vi "MongoDB.CreateIndex.vi"(8 "error in (no error)":errorcluster, 10 "keyNames":string[](array[string]), 11 "MongoDB.Collection in":refnum<class "MongoDB.Collection.lvclass">) -> (0 "error out":errorcluster, 2 "Result":T1, 3 "MongoDB.Collection out":refnum<class "MongoDB.Collection.lvclass">)   [LabVIEW 2014, in "MongoDB.Collection.lvclass"]
uses:
  MongoDB.Collection.lvclass
  MongoDB.Collection.lvclass/MongoDB.Collection.ctl
  C:/Users/Richard/Documents/GitHub/mongo-labview-driver/CSharp/bin/MongoDB.Driver.Legacy.dll
  CSharp/bin/MongoDB.Driver.Legacy.dll
  C:/Users/Richard/Documents/GitHub/mongo-labview-driver/CSharp/bin/MongoDB.Driver.Core.dll
  CSharp/bin/MongoDB.Driver.Core.dll
  C:/Users/Richard/Documents/GitHub/mongo-labview-driver/CSharp/bin/MongoDB.Bson.dll
  CSharp/bin/MongoDB.Bson.dll
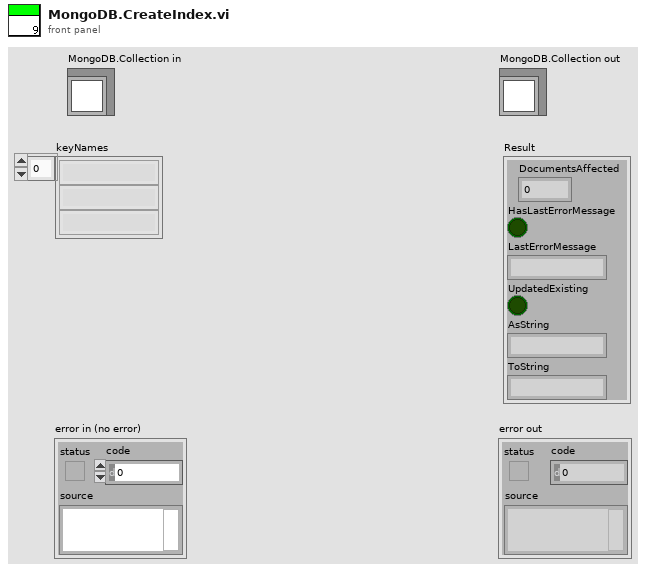
[diagram p1: front panel]
types:
  T1 = cluster{"DocumentsAffected":i64, "HasLastErrorMessage":bool, "LastErrorMessage":string, "UpdatedExisting":bool, "AsString":string, "ToString":string}
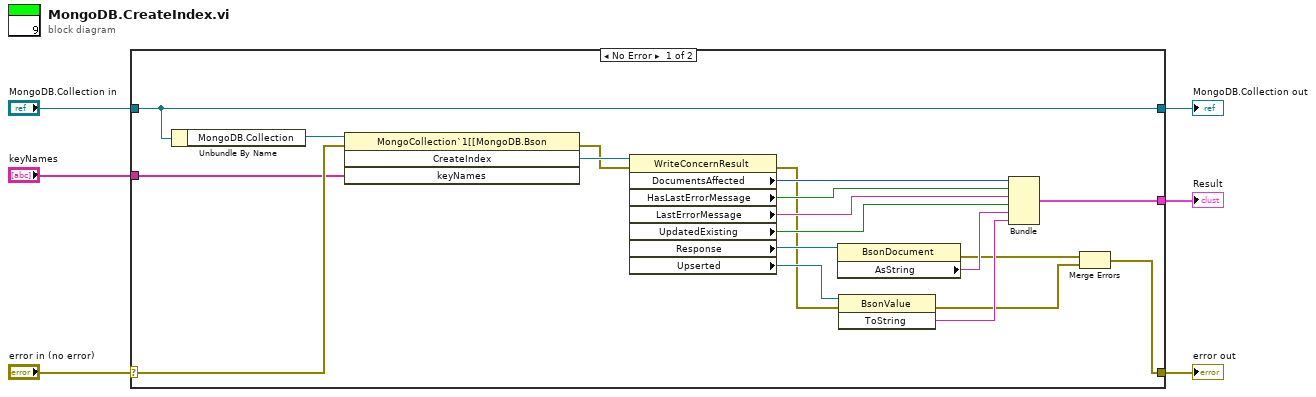
[diagram p0: block diagram]
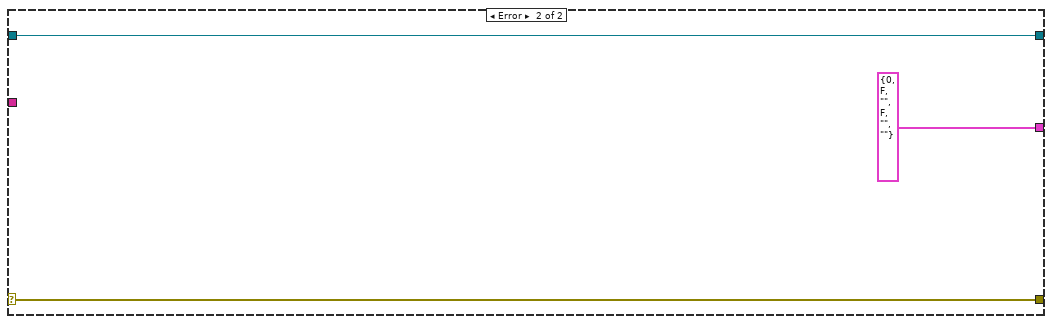
[diagram p2: hidden frame]
diagram:
  n1 = case shown="No Error" "error in (no error)" {
    selector: "error in (no error)" -> [w23 w28]
    tunnel: [w8 w28] -> w5
    tunnel: [w25 w27] -> w3
    tunnel: "MongoDB.Collection in" -> [w25 w27]
    tunnel: "keyNames" -> [w22 _]
    tunnel: [w7 T1 {"DocumentsAffected"=0, "HasLastErrorMessage"=FALSE, "LastErrorMessage"="", "UpdatedExisting"=FALSE, "AsString"="", "ToString"=""}] -> w1
    frame No Error {
      n2 = Unbundle By Name(w25) -> ("MongoDB.Collection"=w24:refnum<k24>)
      n3 = invoke class="MongoCollection`1[[MongoDB.Bson" method="CreateIndex"(reference=w24, error in=w23, "keyNames"=w22) -> (error out=w20:errorcluster, "CreateIndex"=w21:refnum<k24>)  [unwired: 1 in, 2 out]
      n4 = property class="WriteConcernResult"(reference=w21, error in=w20) -> (error out=w12:errorcluster, "DocumentsAffected"=w19:i64, "HasLastErrorMessage"=w18:bool, "LastErrorMessage"=w17:string, "UpdatedExisting"=w16:bool, "Response"=w15:refnum<k24>, "Upserted"=w13:refnum<k24>)  [unwired: 1 out]
      n5 = property class="BsonDocument"(reference=w15) -> (error out=w10:errorcluster, "AsString"=w14:string)  [unwired: 1 in, 1 out]
      n6 = invoke class="BsonValue" method="ToString"(reference=w13, error in=w12) -> (error out=w9:errorcluster, "ToString"=w11:string)  [unwired: 1 in, 1 out]
      n7 = Bundle("DocumentsAffected"=w19, "HasLastErrorMessage"=w18, "LastErrorMessage"=w17, "UpdatedExisting"=w16, "AsString"=w14, "ToString"=w11) -> (w7:T1)  [unwired: 1 in]
      n8 = Merge Errors(w10, w9) -> (w8:errorcluster)
    }
    frame Error {
    }
  }
  "error out" <- w5
  "MongoDB.Collection out" <- w3
  "Result" <- w1
